vi "Untitled 1.vi"() -> ()   [LabVIEW 2016]
panel:
  in  "Frequency 2":dbl=10.1 caption="Frequency"
  in  "Amplitude 2":dbl=1.0 caption="Amplitude"
  in  "Phase 2":dbl caption="Phase"
  in  "Phase":dbl
  in  "Amplitude":dbl=1.0
  in  "Frequency":dbl=10.1
  in  "stop (F)":bool
  out "Waveform Graph":dbl[](graph)
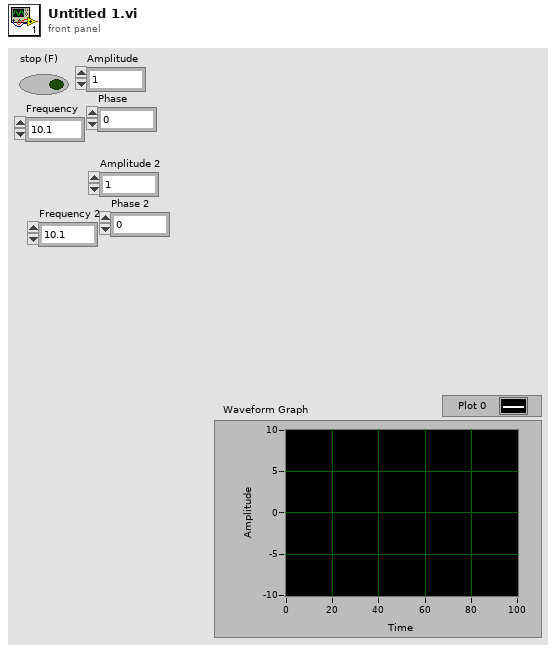
[diagram p1: front panel]
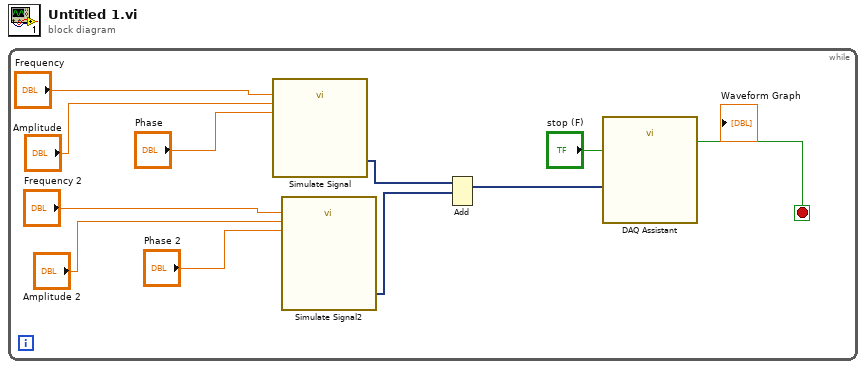
[diagram p0: block diagram]
diagram:
  n1 = while {
    stop <- w10 stop-if-true
    n2 = call "Simulate Signal"("Frequency"="Frequency", "Amplitude"="Amplitude", "Phase"="Phase") -> ("Sine"=w3:dynamicdata)  [unwired: 11 in, 1 out]
    n3 = call "Simulate Signal2"("Frequency"="Frequency 2", "Amplitude"="Amplitude 2", "Phase"="Phase 2") -> ("Sine"=w2:dynamicdata)  [unwired: 11 in, 1 out]
    n4 = Add(1:w2, 2:w3) -> (0:w1:dynamicdata)  [unwired: 1 in, 1 out]
    n5 = call "DAQ Assistant"("data"=w1, "stop (F)"="stop (F)") -> ("stopped"=w10:bool)  [unwired: 15 in, 2 out]
  }
